vi "test_Remove Scalar Input Channels.vi"(8 "error in (no error)":errorcluster, 11 "TestCase in":refnum<class "FPGA Addon Adding Channel Items Unit Tests.lvclass">=refnum) -> (0 "error out":errorcluster, 3 "TestCase out":refnum<class "FPGA Addon Adding Channel Items Unit Tests.lvclass">)   [LabVIEW 2019, in "FPGA Addon Adding Channel Items Unit Tests.lvclass"]
uses:
  FPGA Addon Adding Channel Items Unit Tests.lvclass
  <vilib>/addons/_JKI Toolkits/VI Tester/TestCase.llb/TestCase.lvclass
  <vilib>/NI VeriStand/Custom Device Tools/Custom Device Utility Library/Custom Device Utility Library.lvlib
  Addon/Addon Shared/SubVIs/Constants.vi
  Addon/Addon Shared/FPGA Addon Shared.lvlib
  <vilib>/NI/NI VeriStand Advanced SysDef API/SysDef API/Advanced System Definition.lvlib
  <vilib>/NI VeriStand/Custom Device Tools/Custom Device Utility Library/NI VeriStand - Search for Item by GUID.vi
  Addon/Addon System Explorer/FPGA Addon System Explorer.lvlib
  <vilib>/NI/NI VeriStand Advanced SysDef API/_SubVIs/SysDef.Search.GUIDs.vi
  <vilib>/NI VeriStand/Custom Device API/Custom Device Item Ref.ctl
  <vilib>/NI VeriStand/Custom Device API/Custom Device API.lvlib
  Addon/Addon System Explorer/Types/SE UI Cluster.ctl
panel:
  out "GUIDs":string[](array[string])
  in  "remove":bool
  in  "add":bool
  out "Names":string[](array[string])
  in  "Available Registers":i32[](listbox)
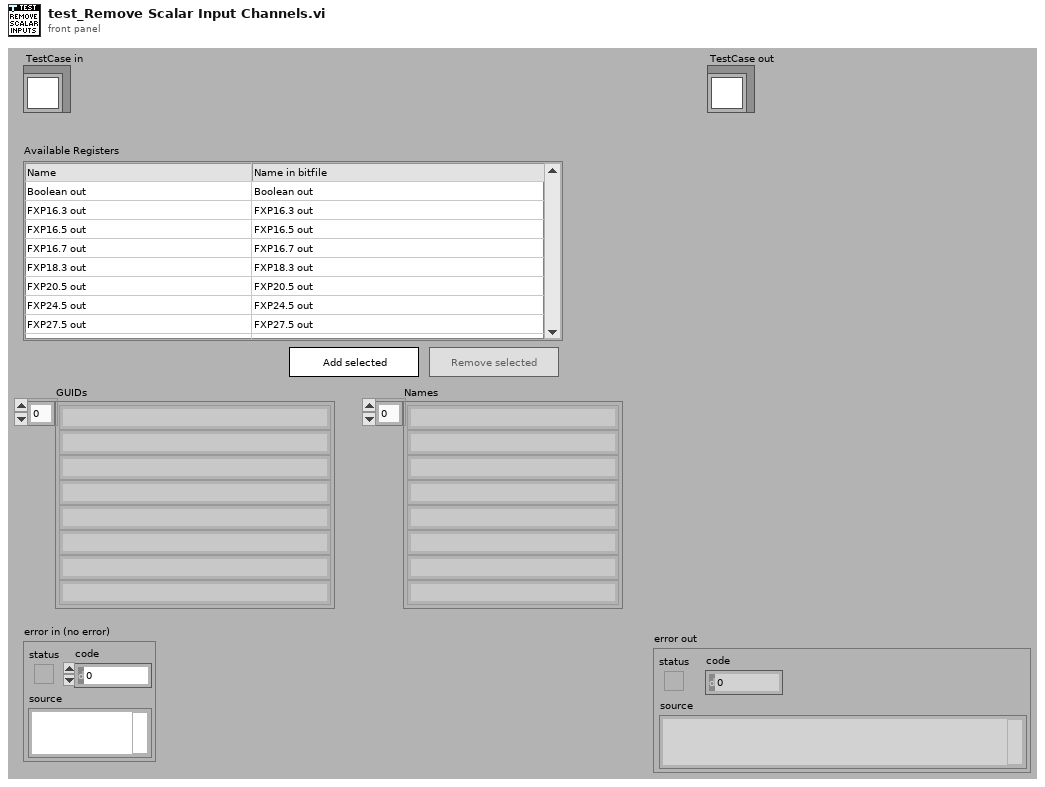
[diagram p1: front panel]
types:
  T1 = typedef "FPGA Addon System Explorer.lvlib/SE UI Cluster.ctl" = cluster{"Node Ptr":T2, "Add":refnum<vi>, "Remove":refnum<vi>, "Registers ListBox":refnum<vi>}
  T2 = typedef "Custom Device API.lvlib/Custom Device Item Ref.ctl" = u64
  T3 = typedef "Advanced System Definition.lvlib/TreeItem.Info.ctl" = cluster{"Name":string, "Description":string, "GUID":string, "Is Channel":bool, "Channel":T4, "Is Waveform":bool, "Waveform":T6}
  T4 = typedef "Custom Device API.lvlib/Custom Device Channel.ctl" = cluster{"Type":T5, "Units":string, "Default Value":dbl, "Faultable":bool, "Scalable":bool}
  T5 = typedef "Custom Device API.lvlib/Custom Device Channel Type.ctl" = enum16{"Input", "Output"}
  T6 = typedef "Custom Device API.lvlib/Custom Device Waveform.ctl" = cluster{"Data Type":T7, "Units":string}
  T7 = typedef "Custom Device API.lvlib/Custom Device Waveform DataType.ctl" = enum16{"Double", "Complex Double"}
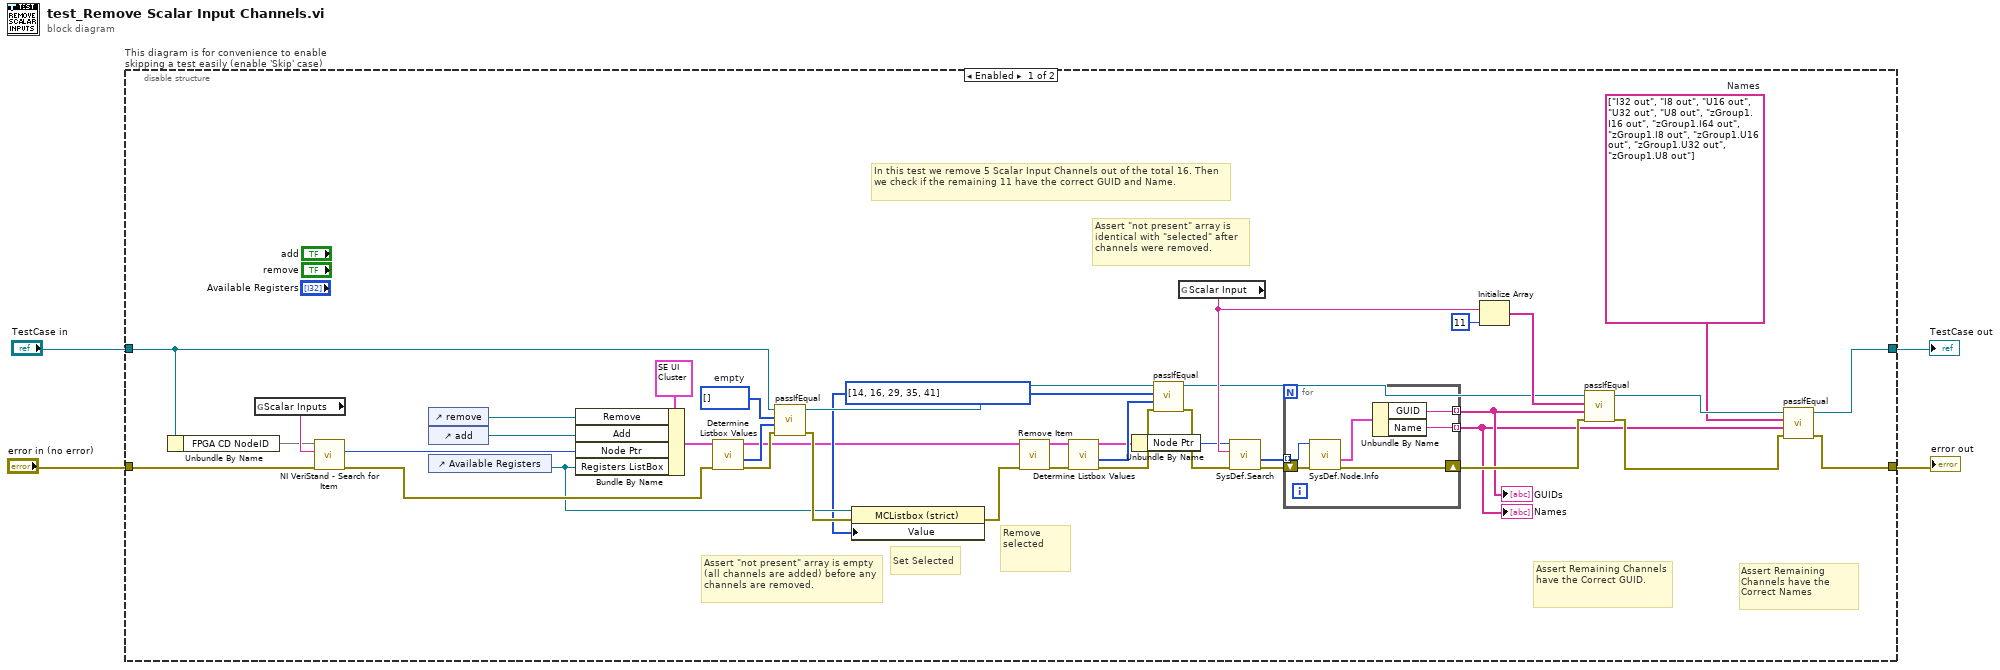
[diagram p0: block diagram]
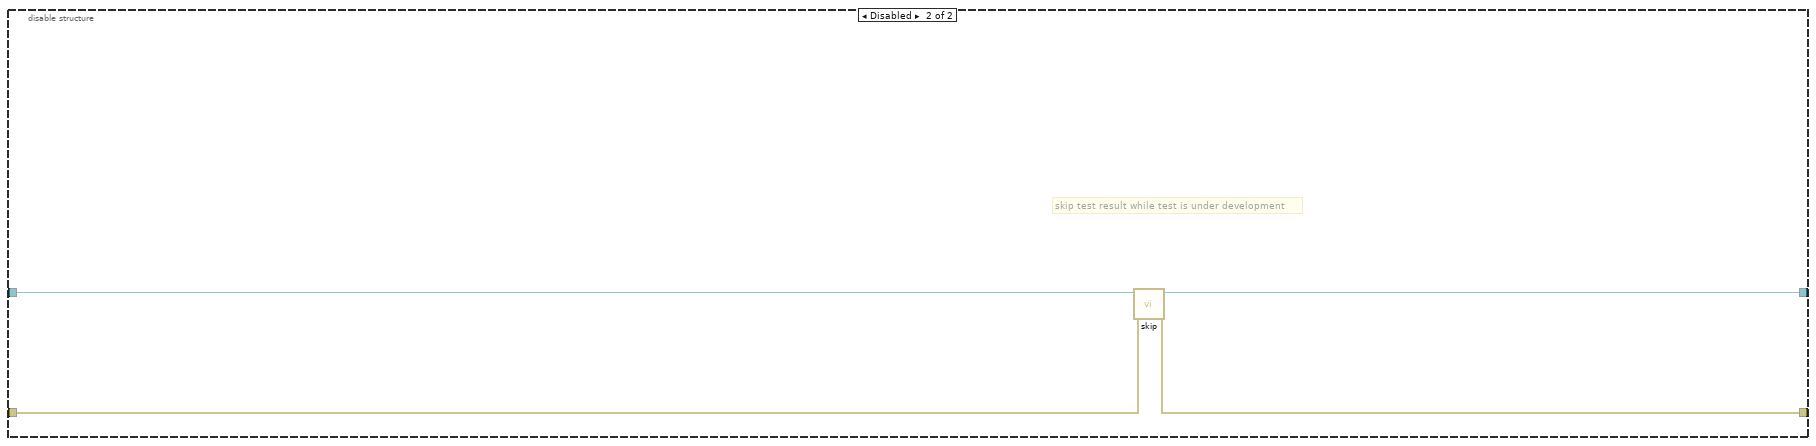
[diagram p2: hidden frame]
diagram:
  n1 = disable-structure "This diagram is for convenience to enable skipping a test easily (enable 'Skip' case)" shown="Enabled" {
    disable-tunnel: "TestCase in" -> [w25 w54]
    disable-tunnel: [w35 w52] -> w1
    disable-tunnel: [w34 w53] -> w3
    disable-tunnel: "error in (no error)" -> [w33 w51]
    frame Enabled {
      w26 = i32[] []  # empty
      w36 = string[] ["I32 out", "I8 out", "U16 out", "U32 out", "U8 out", "zGroup1.I16 out", "zGroup1.I64 out", "zGroup1.I8 out", "zGroup1.U16 out", "zGroup1.U32 out", "zGroup1.U8 out"]  # Names
      w13 = i32[] [14, 16, 29, 35, 41] ("selected")
      # "Remove selected"
      # "Set Selected"
      # "Assert \"not present\" array is empty (all channels are added) before any channels are removed."
      # "Assert \"not present\" array is identical with \"selected\" after channels were removed."
      # "In this test we remove 5 Scalar Input Channels out of the total 16. Then we check if the remaining 11 have the correct GUID and Name."
      # "Assert Remaining Channels have the Correct Names"
      # "Assert Remaining Channels have the Correct GUID."
      n2 = Unbundle By Name(w25) -> ("FPGA CD NodeID"=w32)
      n3 = global read "Constants.vi" "Scalar Inputs"() -> (w44:string)
      n4 = call-poly <vilib>:"NI VeriStand - Search for Item.vi"("error in"=w33, "Item GUID"=w44, "Section Ref in"=w32) -> ("error out"=w17:errorcluster, "Item Ref"=w21:T2)  [unwired: 5 in, 2 out]
      n5 = control-ref of="remove"() -> (w19:refnum<vi>)
      n6 = control-ref of="add"() -> (w18:refnum<vi>)
      n7 = control-ref of="Available Registers"() -> (w14:refnum<vi>)
      n8 = Bundle By Name(cluster=T1 {"Node Ptr"=18446744073709551615, "Add"=refnum, "Remove"=refnum, "Registers ListBox"=refnum} ("SE UI cluster in"), "Remove"=w19, "Add"=w18, "Node Ptr"=w21, "Registers ListBox"=w14) -> (w23:T1)
      n9 = call "Determine Listbox Values.vi"("error in (no error)"=w17, "SE UI cluster in"=w23) -> ("error out"=w16:errorcluster, "Not imported item Indexes"=w20:i32[], "SE UI cluster out"=w8:T1)  [unwired: 6 in, 1 out]
      n10 = call-dynamic "passIfEqual.vi"("error in (no error)"=w16, "y"=w20, "x"=w26, "TestCase in"=w25) -> ("error out"=w15:errorcluster, "TestCase out"=w24:refnum<class "FPGA Addon Adding Channel Items Unit Tests.lvclass">)  [unwired: 6 in]
      n11 = property class="MCListbox (strict)"(reference=w14, error in=w15, "Value"=w13) -> (error out=w9:errorcluster)  [unwired: 1 out]
      n12 = call "Remove Item.vi"("error in (no error)"=w9, "SE UI cluster in"=w8) -> ("error out"=w12:errorcluster, "SE UI cluster out"=w11:T1)  [unwired: 7 in, 1 out]
      n13 = call "Determine Listbox Values.vi"("error in (no error)"=w12, "SE UI cluster in"=w11) -> ("error out"=w7:errorcluster, "Not imported item Indexes"=w10:i32[], "SE UI cluster out"=w6:T1)  [unwired: 6 in, 1 out]
      n14 = Unbundle By Name(w6) -> ("Node Ptr"=w5:T2)
      n15 = call-dynamic "passIfEqual.vi"("error in (no error)"=w7, "y"=w10, "x"=w13, "TestCase in"=w24) -> ("error out"=w28:errorcluster, "TestCase out"=w27:refnum<class "FPGA Addon Adding Channel Items Unit Tests.lvclass">)  [unwired: 6 in]
      n16 = global read "Constants.vi" "Scalar Input"() -> (w30:string)
      n17 = call-poly <vilib>:"SysDef.Search.vi"("error in (no error)"=w28, "GUID"=w30, "nodeID"=w5) -> ("error out"=w43:errorcluster, "Values Out"=w42:u64[])  [unwired: 5 in, 2 out]
      n18 = for {
        tunnel: w42 -> [w47] mode=indexing
        tunnel: [w45] -> w37 mode=indexing
        tunnel: [w46] -> w39 mode=indexing
        shift-right: [w49] -> w40
        shift-left: w43 -> [w50]
        n19 = call <vilib>:"SysDef.Node.Info.vi"("error in (no error)"=w50, "nodeID"=w47) -> ("error out"=w49:errorcluster, "Item Info"=w48:T3)  [unwired: 6 in, 2 out]
        n20 = Unbundle By Name(w48) -> ("GUID"=w46:string, "Name"=w45:string)
      }
      "Names" <- w37
      "GUIDs" <- w39
      n21 = Initialize Array(w30, 11 ("dimension size")) -> (w31:string[])
      n22 = call-dynamic "passIfEqual.vi"("error in (no error)"=w40, "y"=w39, "x"=w31, "TestCase in"=w27) -> ("error out"=w41:errorcluster, "TestCase out"=w38:refnum<class "FPGA Addon Adding Channel Items Unit Tests.lvclass">)  [unwired: 6 in]
      n23 = call-dynamic "passIfEqual.vi"("error in (no error)"=w41, "y"=w37, "x"=w36, "TestCase in"=w38) -> ("error out"=w34:errorcluster, "TestCase out"=w35:refnum<class "FPGA Addon Adding Channel Items Unit Tests.lvclass">)  [unwired: 6 in]
    }
    frame Disabled {
      # "skip test result while test is under development"
      n24 = call <vilib>:"skip.vi"("error in (no error)"=w51, "TestCase in"=w54) -> ("error out"=w53:errorcluster, "TestCase out"=w52:refnum<class "TestCase.lvclass">)  [unwired: 8 in]
    }
  }
  "error out" <- w3
  "TestCase out" <- w1
